vi "RTS Macro Get Data.vi"(8 "Error In":errorcluster, 10 "Path":path, 11 "Full Refrigeration Data":T1) -> (0 "Error Out":errorcluster, 3 "Refrigeration Full Data Output":T1, 5 "all rows":string[][](array[string]), 7 "deleted portion":string[][](array[string]))   [LabVIEW 2016]
uses:
  Type Definitions/RTS Macro Full Data.ctl
  <vilib>/Utility/file.llb/Read Delimited Spreadsheet (string).vi
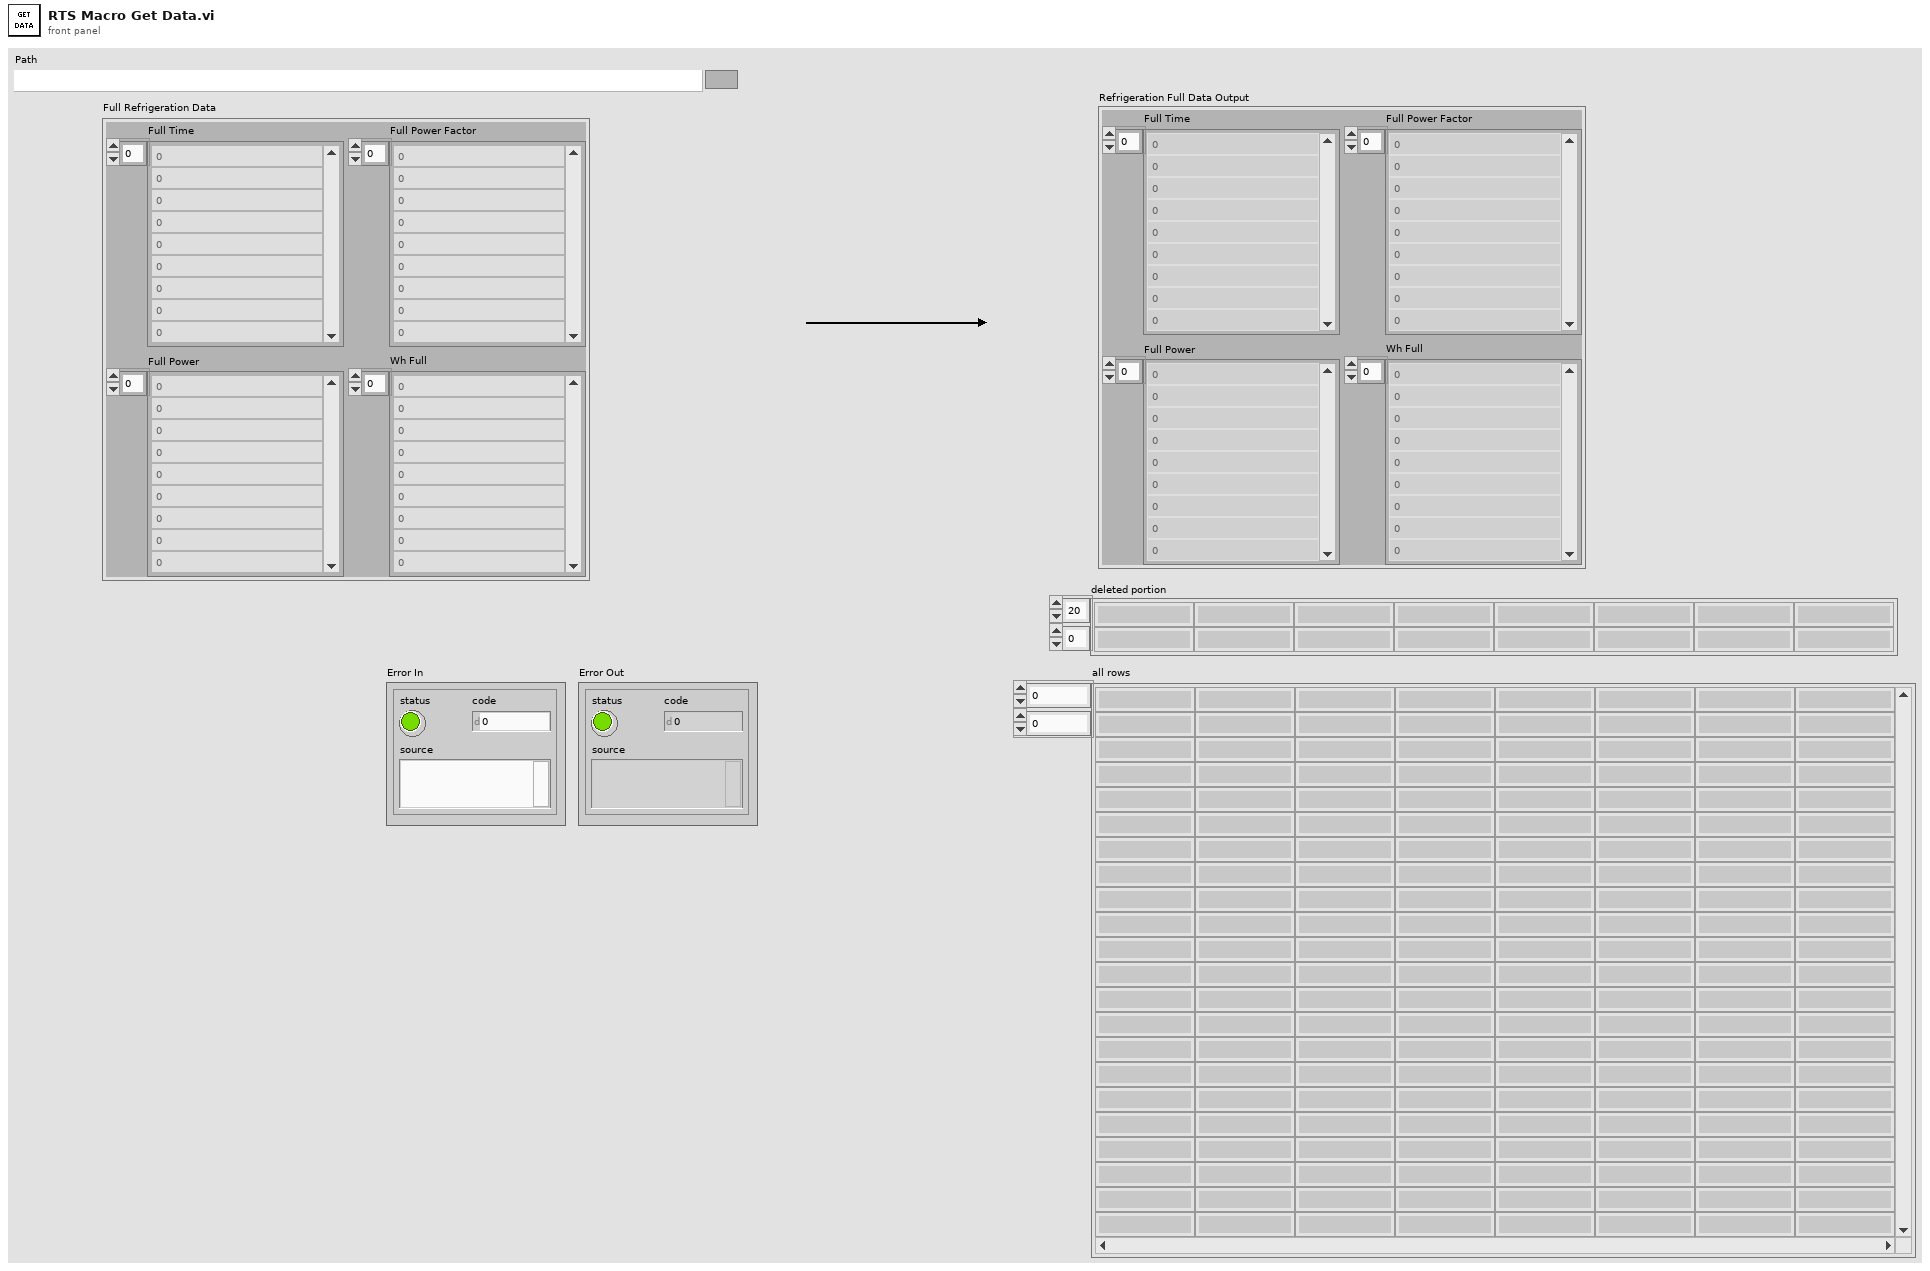
[diagram p1: front panel]
types:
  T1 = typedef "RTS Macro Full Data.ctl" = cluster{"Full Time":dbl[], "Full Power Factor":dbl[], "Full Power":dbl[], "Wh Full":dbl[]}
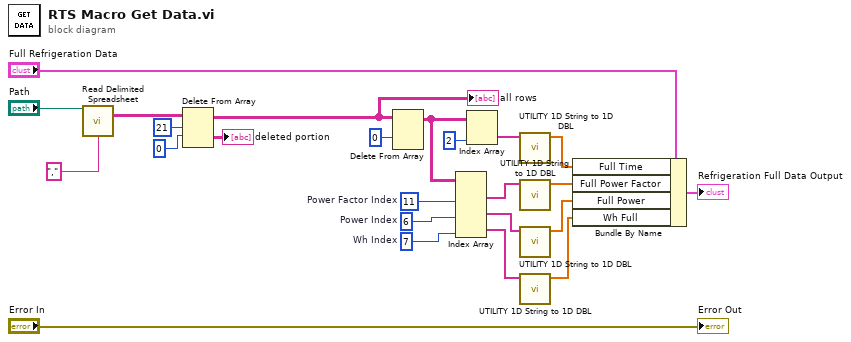
[diagram p0: block diagram]
diagram:
  w16 = 7  # Wh Index
  w15 = 6  # Power Index
  w8 = 11  # Power Factor Index
  n1 = call-poly <vilib>:"Read Delimited Spreadsheet.vi"("file path (dialog if empty)"="Path", "delimiter (\\t)"="," ("delimiter (\\t)")) -> ("all rows"=w4:string[][])  [unwired: 8 in, 5 out]
  n2 = Delete From Array(array=w4, length=21, index (row)=0) -> (deleted portion=→"deleted portion":string[][], array with subset deleted=w12:string[][])  [unwired: 1 in]
  "all rows" <- w12
  n3 = Delete From Array(array=w12, index (row)=0) -> (array with subset deleted=w14:string[][])  [unwired: 2 in, 1 out]
  n4 = Index Array(array=w14, index (col) #1=w8, index (col) #2=w15, index (col) #3=w16) -> (element #1=w9:string[], element #2=w17:string[], element #3=w18:string[])  [unwired: 3 in]
  n5 = Index Array(array=w14, index (col)=2 ("disabled index (col)")) -> (element=w11:string[])  [unwired: 1 in]
  n6 = call "UTILITY 1D String to 1D DBL.vi"("Save Data"=w11) -> ("DBL"=w20:dbl[])  [unwired: 10 in]
  n7 = call "UTILITY 1D String to 1D DBL.vi"("Save Data"=w9) -> ("DBL"=w21:dbl[])  [unwired: 10 in]
  n8 = call "UTILITY 1D String to 1D DBL.vi"("Save Data"=w17) -> ("DBL"=w22:dbl[])  [unwired: 10 in]
  n9 = call "UTILITY 1D String to 1D DBL.vi"("Save Data"=w18) -> ("DBL"=w23:dbl[])  [unwired: 10 in]
  n10 = Bundle By Name(cluster="Full Refrigeration Data", "Full Time"=w20, "Full Power Factor"=w21, "Full Power"=w22, "Wh Full"=w23) -> (→"Refrigeration Full Data Output":T1)
  "Error Out" <- "Error In"
